vi "ACLR auto setup.vi"(8 "error in (no error)":errorcluster, 10 "Setup":T1(ring), 11 "SA-FSW in":refnum<class "SA-FSW.lvclass">) -> (0 "error out":errorcluster, 3 "SA-FSW out":refnum<class "SA-FSW.lvclass">)   [LabVIEW 2020, in "SA-FSW.lvclass"]
uses:
  SA-FSW.lvclass
  C:/Sandbox/Git_Sandbox/WiSpry Test Framework source code (LV20)/WiSpry Test Framework/Instruments/Instrument.lvclass
  C:/Sandbox/Git_Sandbox/WiSpry Test Framework source code (LV20)/WiSpry Test Framework/Instruments/Spectrum Analyzer/Spectrum Analyzer.lvclass
  Instrument.lvclass/Instrument.ctl
  <vilib>/Utility/error.llb/whitespace.ctl
  Spectrum Analyzer.lvclass/Spectrum Analyzer.ctl
  Instrument.lvclass
  Spectrum Analyzer.lvclass
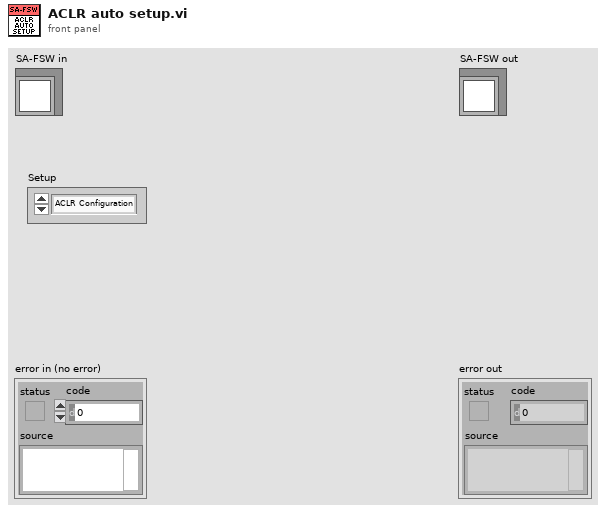
[diagram p1: front panel]
types:
  T1 = enum16{"ACLR Configuration", "Reference Level", "Both"}
  T2 = typedef "whitespace.ctl" = u16
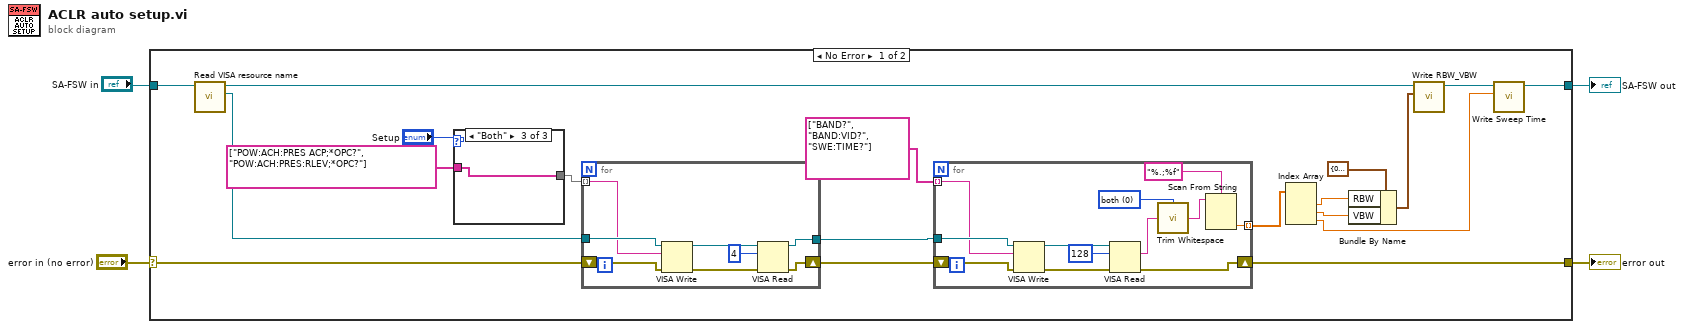
[diagram p0: block diagram]
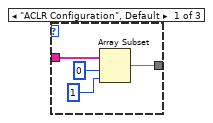
[diagram p2: hidden frame]
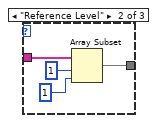
[diagram p3: hidden frame]
diagram:
  n1 = case shown="No Error" "error in (no error)" {
    selector: "error in (no error)" -> [w20 w54]
    tunnel: [w13 w54] -> w3
    tunnel: "SA-FSW in" -> [w23 w53]
    tunnel: [w6 w53] -> w1
    frame No Error {
      n2 = call "Read VISA resource name.vi"("Instrument in"=w23) -> ("VISA resource name"=w18:refnum<visa-resource-name>, "Instrument out"=w17:refnum<class "SA-FSW.lvclass">)  [unwired: 9 in]
      n3 = case shown="\"Both\"" "Setup" {
        tunnel: string[] ["POW:ACH:PRES ACP;*OPC?", "POW:ACH:PRES:RLEV;*OPC?"] -> [w47 w51 w52]
        tunnel: [w44 w48 w52] -> w19
        frame "ACLR Configuration", Default {
          n4 = Array Subset(array=w47, index=0, length=1) -> (w44:string[])
        }
        frame "Reference Level" {
          n5 = Array Subset(array=w51, index=1, length=1) -> (w48:string[])
        }
        frame "Both" {
        }
      }
      n6 = for {
        shift-right: [w40] -> w16
        shift-left: w20 -> [w43]
        tunnel: w19 -> [w41] mode=indexing
        tunnel: w18 -> [w42]
        tunnel: [w36] -> w15
        n7 = VISA Write(VISA resource name=w42, write buffer=w41, error in (no error)=w43) -> (VISA resource name out=w38:refnum<visa-resource-name>, error out=w39:errorcluster)  [unwired: 1 out]
        n8 = VISA Read(VISA resource name=w38, byte count=u32 4, error in (no error)=w39) -> (VISA resource name out=w36:refnum<visa-resource-name>, error out=w40:errorcluster)  [unwired: 2 out]
      }
      n9 = for {
        shift-right: [w32] -> w13
        shift-left: w16 -> [w35]
        tunnel: string[] ["BAND?", "BAND:VID?", "SWE:TIME?"] -> [w33] mode=indexing
        tunnel: w15 -> [w34]
        tunnel: [w24] -> w10 mode=indexing
        w27 = T2 0 items=["both", "start of string", "end of string"] ("location (both)")
        n10 = VISA Write(VISA resource name=w34, write buffer=w33, error in (no error)=w35) -> (VISA resource name out=w30:refnum<visa-resource-name>, error out=w31:errorcluster)  [unwired: 1 out]
        n11 = VISA Read(VISA resource name=w30, byte count=u32 128, error in (no error)=w31) -> (read buffer=w28:string, error out=w32:errorcluster)  [unwired: 2 out]
        n12 = call <vilib>:"Trim Whitespace.vi"("string"=w28, "location (both)"=w27) -> ("trimmed string"=w26:string)
        n13 = Scan From String(format string="%.;%f", input string=w26) -> (output 1=w24:dbl)  [unwired: 3 in, 3 out]
      }
      n14 = Index Array(array=w10) -> (element #1=w9:dbl, element #2=w8:dbl, element #3=w5:dbl)  [unwired: 3 in]
      n15 = Bundle By Name(cluster=cluster{"RBW":dbl, "VBW":dbl} {"RBW"=0.0, "VBW"=0.0} ("RBW/VBW"), "RBW"=w9, "VBW"=w8) -> (w11:cluster{"RBW":dbl, "VBW":dbl})
      n16 = call "Write RBW_VBW.vi"("RBW/VBW"=w11, "Spectrum Analyzer in"=w17) -> ("Spectrum Analyzer out"=w7:refnum<class "SA-FSW.lvclass">)  [unwired: 9 in]
      n17 = call "Write Sweep Time.vi"("Sweep Time"=w5, "Spectrum Analyzer in"=w7) -> ("Spectrum Analyzer out"=w6:refnum<class "SA-FSW.lvclass">)  [unwired: 9 in]
    }
    frame Error {
    }
  }
  "error out" <- w3
  "SA-FSW out" <- w1
